vi "ziTicksToS_single.vi"(3 "Error In":errorcluster, 4 "Timestamp(ticks)":u64, 5 "Handle In":T1 {"Handle" format="0x%08x"; "Conn" format="0x%08x"}) -> (0 "Error Out":errorcluster, 1 "Timestamp(s)":dbl, 2 "Handle Out":T1 {"Handle" format="0x%08x"; "Conn" format="0x%08x"})   [LabVIEW 2018, in "Zurich Instruments LabOne.lvlib"]
uses:
  Zurich Instruments LabOne.lvlib
  ziTypeHandle.ctl
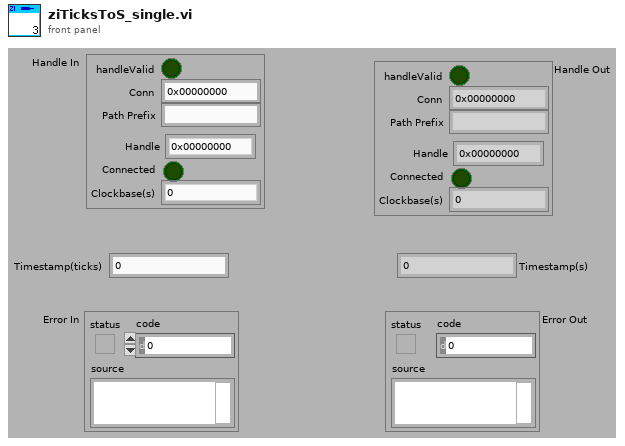
[diagram p1: front panel]
types:
  T1 = typedef "Zurich Instruments LabOne.lvlib/ziTypeHandle.ctl" = cluster{"handleValid":bool, "Conn":u64, "Path Prefix":string, "Handle":u64, "Connected":bool, "Clockbase(s)":dbl}
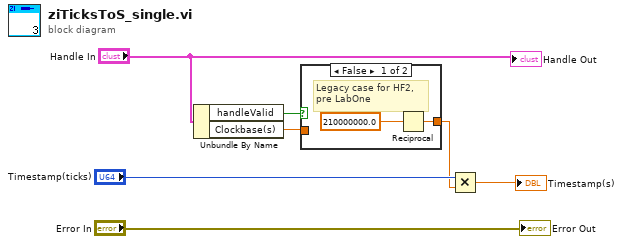
[diagram p0: block diagram]
diagram:
  n1 = Unbundle By Name("Handle In") -> ("handleValid"=w3:bool, "Clockbase(s)"=w2:dbl)
  n2 = case shown="False" w3 {
    tunnel: [w8 w10] -> w5
    tunnel: w2 -> [_ w10]
    frame False {
      # "Legacy case for HF2, \npre LabOne"
      n3 = Reciprocal(x=210000000.0 ("s")) -> (1/x=w8:dbl)
    }
    frame True {
    }
  }
  n4 = Multiply(x="Timestamp(ticks)", y=w5) -> (x*y=→"Timestamp(s)":dbl)
  "Handle Out" <- "Handle In"
  "Error Out" <- "Error In"
